vi "New Packet from Bytes.vi"(8 "error in (no error)":errorcluster, 10 "Bytes":u8[](array[numeric])) -> (0 "error out":errorcluster, 3 "Packet out":refnum<class "Packet.lvclass">)   [LabVIEW 2020, in "Communication Classes.lvlib" / "Packet.lvclass"]
uses:
  Packet.lvclass
  Packet.lvclass/Packet.ctl
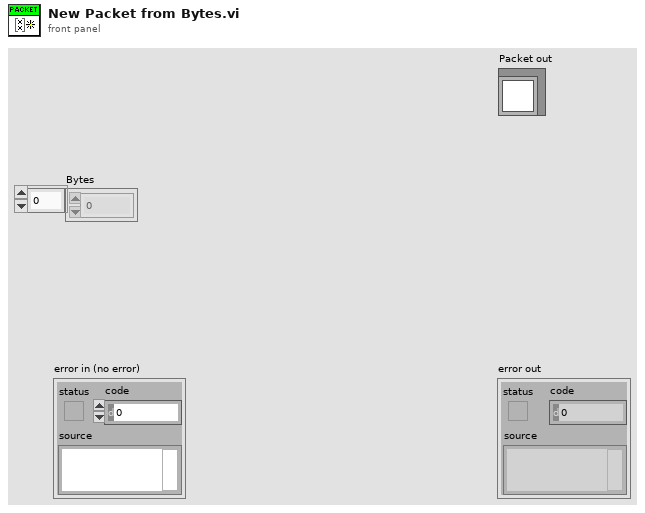
[diagram p1: front panel]
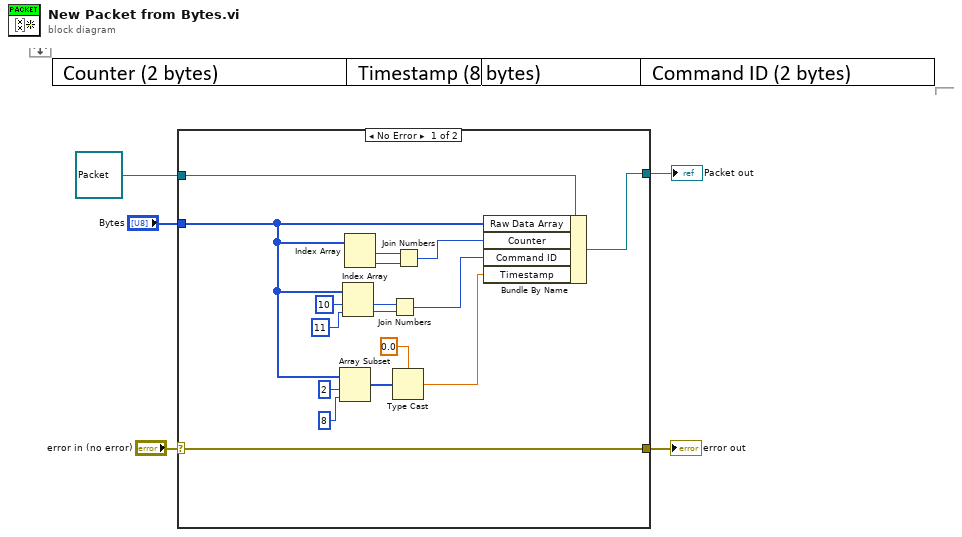
[diagram p0: block diagram]
diagram:
  n1 = case shown="No Error" "error in (no error)" {
    selector: "error in (no error)" -> [w22 w24]
    tunnel: [w22 w24] -> w4
    tunnel: refnum<class "Packet.lvclass"> refnum ("Communication.lvlib:Packet.lvclass") -> [w21 w23]
    tunnel: "Bytes" -> [w11 _]
    tunnel: [w20 w23] -> w1
    frame No Error {
      n2 = Array Subset(array=w11, index=2, length=8 ("index")) -> (w8:u8[])
      n3 = Index Array(array=w11, index #1=10 ("index"), index #2=11 ("index")) -> (element #1=w14:u8, element #2=w13:u8)
      n4 = Index Array(array=w11) -> (element #1=w18:u8, element #2=w19:u8)  [unwired: 2 in]
      n5 = Join Numbers(hi=w14, lo=w13) -> ((hi.lo)=w12:u16)
      n6 = Type Cast(type=0.0, x=w8) -> (*(type *) &x=w6:dbl)
      n7 = Join Numbers(hi=w18, lo=w19) -> ((hi.lo)=w17:u16)
      n8 = Bundle By Name(cluster=w21, "Raw Data Array"=w11, "Counter"=w17, "Command ID"=w12, "Timestamp"=w6) -> (w20:refnum<class "Packet.lvclass">)
    }
    frame Error {
    }
  }
  "error out" <- w4
  "Packet out" <- w1
